vi "Get Default Step from Database.vi"(8 "error in (no error)":errorcluster, 10 "Default Step":string, 11 "Measurement Interface in":refnum<class "Measurement Interface.lvclass">) -> (0 "error out":errorcluster, 2 "Cloned Step":refnum<k7>, 3 "Measurement Interface out":refnum<class "Measurement Interface.lvclass">)   [LabVIEW 2016, in "Measurement Interface.lvlib" / "Measurement Interface.lvclass"]
uses:
  Measurement Interface.lvclass
  Measurement Interface.lvclass/Measurement Interface.ctl
  Plugins/TestStand API Tools (TSAT).lvlibp/Step Actions/TSAT Step Actions.lvlib
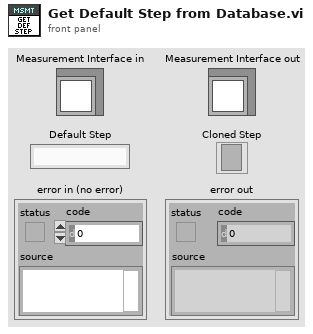
[diagram p1: front panel]
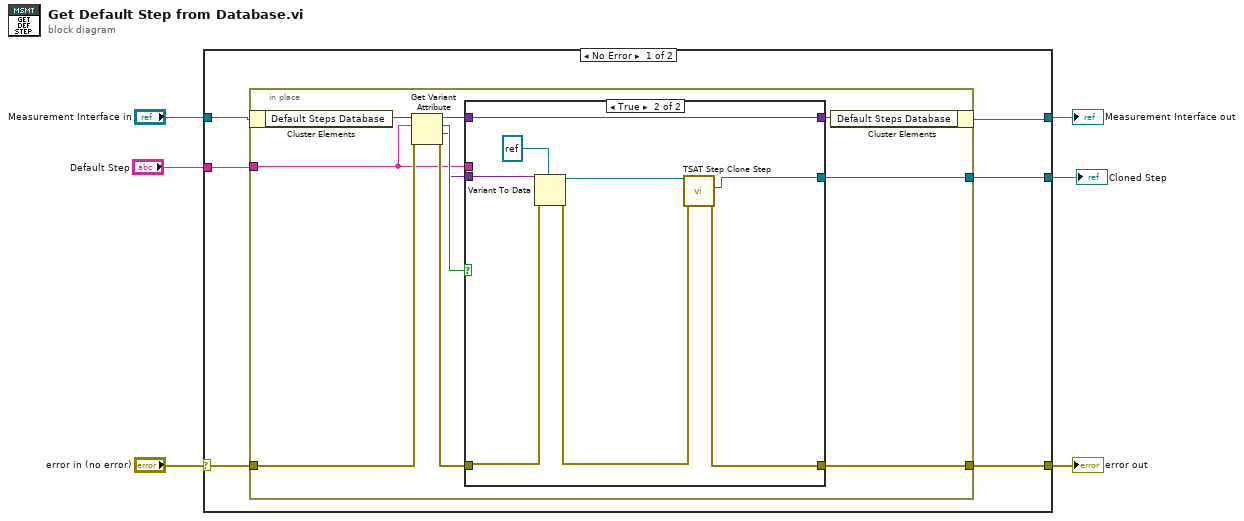
[diagram p0: block diagram]
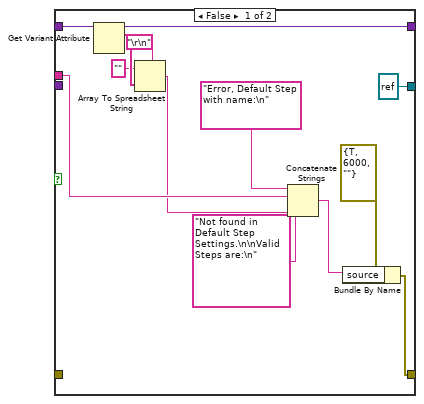
[diagram p2: hidden frame]
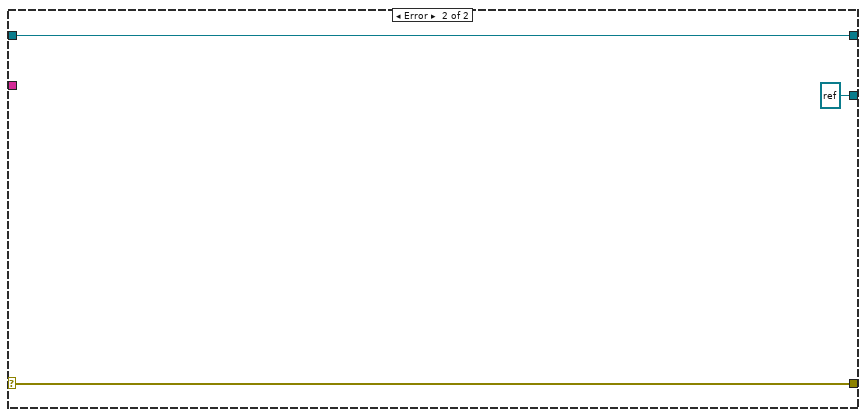
[diagram p3: hidden frame]
diagram:
  n1 = case shown="No Error" "error in (no error)" {
    selector: "error in (no error)" -> [w9 w46]
    tunnel: [w8 w46] -> w5
    tunnel: [w11 w45] -> w3
    tunnel: "Measurement Interface in" -> [w12 w45]
    tunnel: [w10 refnum<k7> refnum ("Cloned Step")] -> w2
    tunnel: "Default Step" -> [w7 _]
    frame No Error {
      n2 = in-place {
        in-place-border: [w17] -> w8
        in-place-border: w9 -> [w21]
        in-place-border: w7 -> [w18]
        in-place-border: [w15] -> w10
        n3 = in-place-cluster #1(w12) -> ("Default Steps Database"=w22:variant)
        n4 = Get Variant Attribute(Variant=w22, name=w18, error in=w21) -> (duplicate Variant=w13:variant, found=w20:bool, value=w16:variant, error out=w19:errorcluster)  [unwired: 1 in]
        n5 = case shown="True" w20 {
          tunnel: w19 -> [_ w37]
          tunnel: w18 -> [w32 _]
          tunnel: [w30 w43] -> w17
          tunnel: w16 -> [_ w40]
          tunnel: [refnum<k7> refnum ("Cloned Step") w42] -> w15
          tunnel: [w27 w41] -> w14
          tunnel: w13 -> [w28 w41]
          frame False {
            n6 = Get Variant Attribute(Variant=w28) -> (duplicate Variant=w27:variant, names=w26:string[])  [unwired: 3 in, 2 out]
            n7 = Array To Spreadsheet String(delimiter (Tab)="\r\n", array=w26, 3:"" ("format string")) -> (spreadsheet string=w23:string)
            n8 = Concatenate Strings("Error, Default Step with name:\n", w32, "Not found in Default Step Settings.\n\nValid Steps are:\n", w23) -> (w34:string)
            n9 = Bundle By Name(cluster=errorcluster {"status"=TRUE, "code"=6000, "source"=""} ("error constant"), "source"=w34) -> (w30:errorcluster)
          }
          frame True {
            n10 = Variant To Data(error in=w37, type=refnum<k7> refnum ("Step Reference"), Variant=w40) -> (data=w38:refnum<k7>, error out=w36:errorcluster)
            n11 = call "TSAT Step Clone Step.vi"("Error In"=w36, "Step In"=w38) -> ("Error Out"=w43:errorcluster, "Cloned Step"=w42:refnum<k7>)  [unwired: 7 in, 1 out]
          }
        }
        n12 = in-place-cluster #1("Default Steps Database"=w14) -> (w11:refnum<class "Measurement Interface.lvclass">)
      }
    }
    frame Error {
    }
  }
  "error out" <- w5
  "Measurement Interface out" <- w3
  "Cloned Step" <- w2
